vi "Reset.vi"(8 "error in (no error)":errorcluster, 11 "VISA resource name":refnum<visa-resource-name>) -> (0 "error out":errorcluster, 3 "VISA resource name out":refnum<visa-resource-name>)   [LabVIEW 2019, in "Lake Shore 325.lvlib"]
doc: "Resets the instrument and then sends a set of default setup commands to the instrument."
uses:
  Lake Shore 325.lvlib
  Instance           2 13Saved   Reset .vi
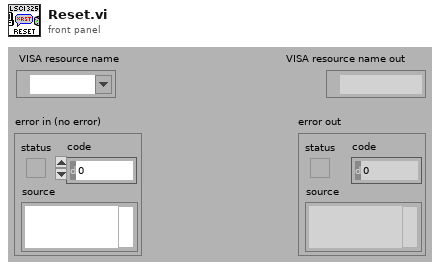
[diagram p1: front panel]
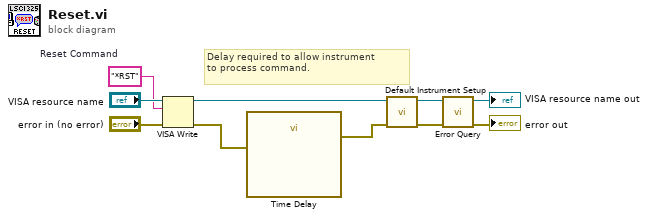
[diagram p0: block diagram]
diagram:
  w8 = "*RST"  # Reset Command
  # "Delay required to allow instrument\nto process command."
  n1 = VISA Write(VISA resource name="VISA resource name", write buffer=w8, error in (no error)="error in (no error)") -> (VISA resource name out=w2:refnum<visa-resource-name>, error out=w3:errorcluster)  [unwired: 1 out]
  n2 = call "Time Delay"("error in (no error)"=w3) -> ("error out"=w1:errorcluster)  [unwired: 10 in]
  n3 = call "Default Instrument Setup.vi"("error in (no error)"=w1, "VISA resource name"=w2) -> ("error out"=w7:errorcluster, "VISA resource name out"=w6:refnum<visa-resource-name>)  [unwired: 8 in]
  n4 = call "Error Query.vi"("error in (no error)"=w7, "VISA resource name"=w6) -> ("error out"=→"error out":errorcluster, "VISA resource name out"=→"VISA resource name out":refnum<visa-resource-name>)  [unwired: 7 in, 1 out]
